vi "LabVIEW_commandline.vi"() -> ()   [LabVIEW 2016]
panel:
  in  "PD Filepath":path=path "D:/PDE Project/PDE Data/Default Data/PD.tdms"
  in  "TC Filepath":path=path "D:/PDE Project/PDE Data/Default Data/TC.tdms"
  in  "PT Filepath":path=path "D:/PDE Project/PDE Data/Default Data/PT.tdms"
  in  "Diluent":string="'N2'"
  in  "Menu Ring":u16(ring) items=["Manual Find", "Use Path"]
  in  "Working Directory":path=path "D:/PDE Project/PDE Data/Default Data/PT.tdms"
  out "text":string="activate python3\npython massflowcalcuator.py"
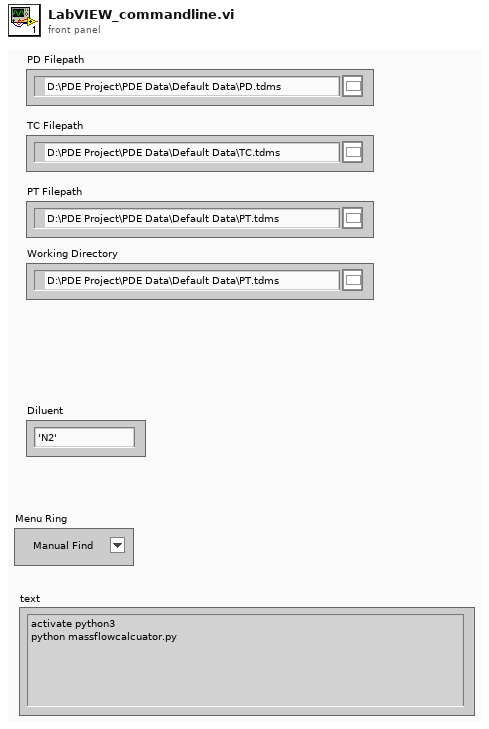
[diagram p1: front panel]
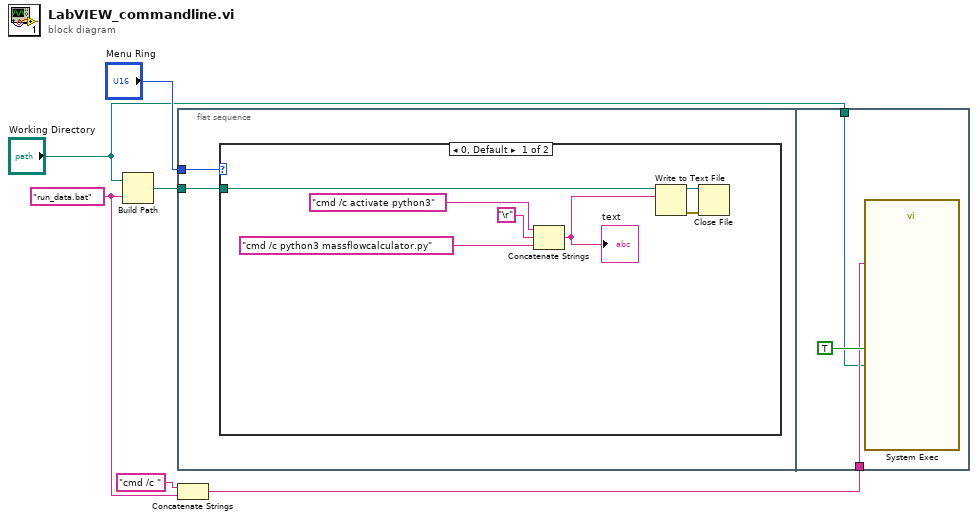
[diagram p0: block diagram]
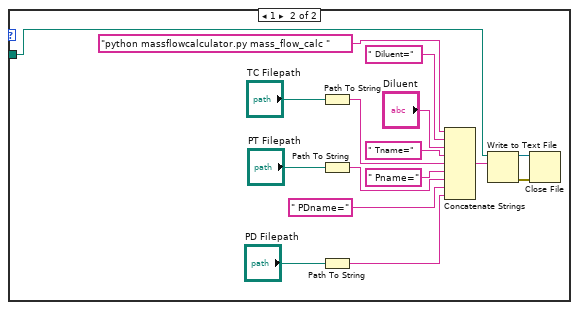
[diagram p2: hidden frame]
diagram:
  w3 = "run_data.bat"
  n1 = Build Path(base path="Working Directory", name or relative path=w3) -> (appended path=w5:path)
  n2 = flat-sequence {
    tunnel: "Menu Ring" -> [w8]
    tunnel: w5 -> [w7]
    tunnel: w4 -> [w33]
    tunnel: "Working Directory" -> [w32]
    frame #0 {
      n3 = case shown="0, Default" w8 {
        tunnel: w7 -> [w9 w17]
        frame 0, Default {
          n4 = Concatenate Strings("cmd /c activate python3" ("text"), "\r", "cmd /c python3 massflowcalculator.py") -> (w10:string)
          "text" <- w10
          n5 = Write to Text File(file (use dialog)=w9, text=w10) -> (refnum out=w14:refnum<file>, error out=w15:errorcluster)  [unwired: 2 in, 1 out]
          n6 = Close File(refnum=w14, error in=w15) -> ()  [unwired: 2 out]
        }
        frame 1 {
          n7 = Path To String(path="TC Filepath") -> (string=w27:string)
          n8 = Path To String(path="PT Filepath") -> (string=w25:string)
          n9 = Path To String(path="PD Filepath") -> (string=w23:string)
          n10 = Concatenate Strings("python massflowcalculator.py mass_flow_calc " ("command line"), " Diluent=", "Diluent", " Tname=" ("string"), w27, " Pname=" ("string"), w25, " PDname=" ("string"), w23) -> (w16:string)
          n11 = Write to Text File(file (use dialog)=w17, text=w16) -> (refnum out=w18:refnum<file>, error out=w19:errorcluster)  [unwired: 2 in, 1 out]
          n12 = Close File(refnum=w18, error in=w19) -> ()  [unwired: 2 out]
        }
      }
    }
    frame #1 {
      n13 = call <vilib>:"System Exec.vi"("wait until completion? (T)"=TRUE, "working directory"=w32, "command line"=w33) -> ()  [unwired: 5 in, 4 out]
    }
  }
  n14 = Concatenate Strings("cmd /c " ("string"), w3) -> (w4:string)
